vi "LFA_Capture.vi"(8 "error in (no error)":errorcluster, 10 "Frames":i32, 11 "LightField Automation in":refnum<class "LightField Automation.lvclass">) -> (0 "error out":errorcluster, 2 "Data":T1(array[cluster]), 3 "LightField Automation out":refnum<class "LightField Automation.lvclass">)   [LabVIEW 2013, in "LightField Automation.lvclass"]
uses:
  LightField Automation.lvclass
  LightField Automation.lvclass/LightField Automation.ctl
  C:/Program Files/Princeton Instruments/LightField/AddInViews/PrincetonInstruments.LightFieldViewV3.dll
  Program Files/Princeton Instruments/LightField/AddInViews/PrincetonInstruments.LightFieldViewV3.dll
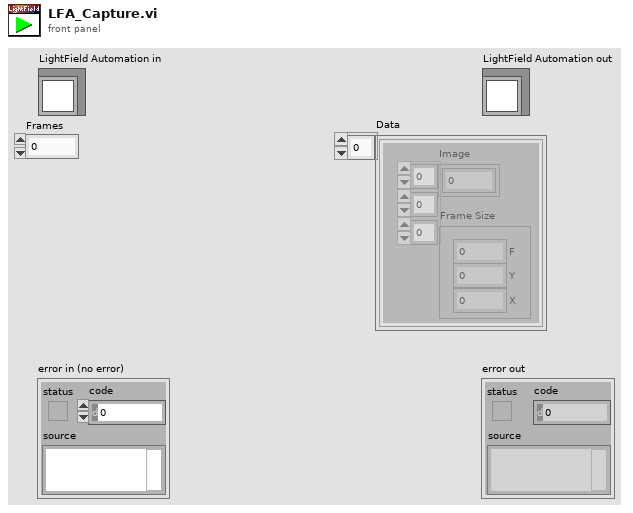
[diagram p1: front panel]
types:
  T1 = cluster{"Image":dbl[][][], "Frame Size":cluster{"F":i32, "Y":i32, "X":i32}}[]
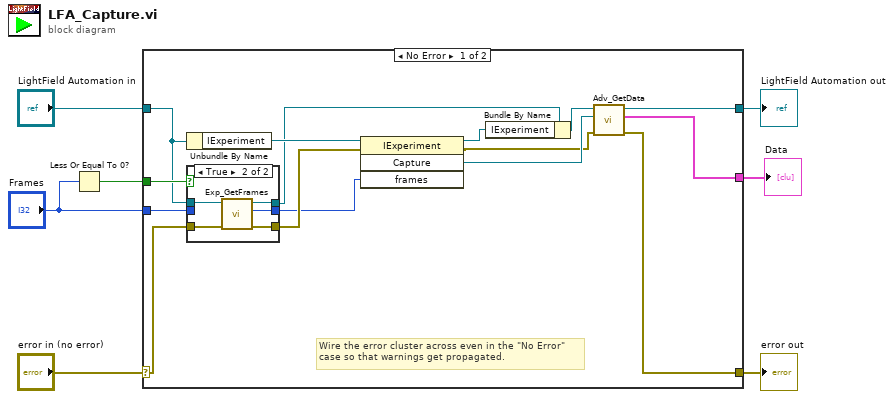
[diagram p0: block diagram]
diagram:
  n1 = Less Or Equal To 0?(x="Frames") -> (x <= 0?=w2:bool)
  n2 = case shown="No Error" "error in (no error)" {
    selector: "error in (no error)" -> [w16 w32]
    tunnel: [w19 w32] -> w6
    tunnel: [w21 w31] -> w4
    tunnel: "LightField Automation in" -> [w15 w31]
    tunnel: [w18 _] -> w3
    tunnel: w2 -> [w17 _]
    tunnel: "Frames" -> [w12 _]
    frame No Error {
      # "Wire the error cluster across even in the \"No Error\"\ncase so that warnings get propagated."
      n3 = Unbundle By Name(w15) -> ("IExperiment"=w22:refnum<k24>)
      n4 = case shown="True" w17 {
        tunnel: w16 -> [w24 w30]
        tunnel: w15 -> [w25 w29]
        tunnel: [w25 w28] -> w10
        tunnel: [w24 w27] -> w14
        tunnel: [w23 w26] -> w13
        tunnel: w12 -> [w23 _]
        frame False {
        }
        frame True {
          n5 = call "Exp_GetFrames.vi"("error in (no error)"=w30, "LightField Automation in"=w29) -> ("error out"=w27:errorcluster, "Frames"=w26:i32, "LightField Automation out"=w28:refnum<class "LightField Automation.lvclass">)  [unwired: 7 in]
        }
      }
      n6 = invoke class="IExperiment" method="Capture"(reference=w22, error in=w14, "frames"=w13) -> (reference out=w8:refnum<k24>, error out=w11:errorcluster, "Capture"=w20:refnum<k24>)  [unwired: 1 in, 1 out]
      n7 = Bundle By Name(cluster=w10, "IExperiment"=w8) -> (w9:refnum<class "LightField Automation.lvclass">)
      n8 = call "Adv_GetData.vi"("error in (no error)"=w11, "IImageDataSet"=w20, "LightField Automation in"=w9) -> ("error out"=w19:errorcluster, "Data"=w18:T1, "LightField Automation out"=w21:refnum<class "LightField Automation.lvclass">)  [unwired: 6 in]
    }
    frame Error {
    }
  }
  "error out" <- w6
  "LightField Automation out" <- w4
  "Data" <- w3
